vi "StrongBandpass.vi"(10 "Frequency":u32, 11 "Numeric":fxp<+/-,24,8>) -> (3 "Output":fxp<+/-,16,4>)   [LabVIEW 2015]
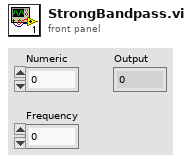
[diagram p1: front panel]
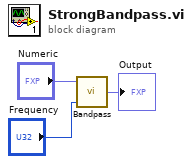
[diagram p0: block diagram]
diagram:
  n1 = call "Bandpass.vi"("Frequency"="Frequency", "Input"="Numeric") -> ("Output"=→"Output":fxp<+/-,24,12>)  [unwired: 3 in]
